vi "temp_Modify Data of First Version.vi"(10 "string":string="V+-V") -> (2 "result string 2":string)   [LabVIEW 2023]
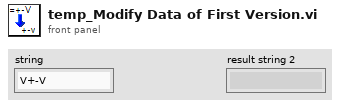
[diagram p1: front panel]
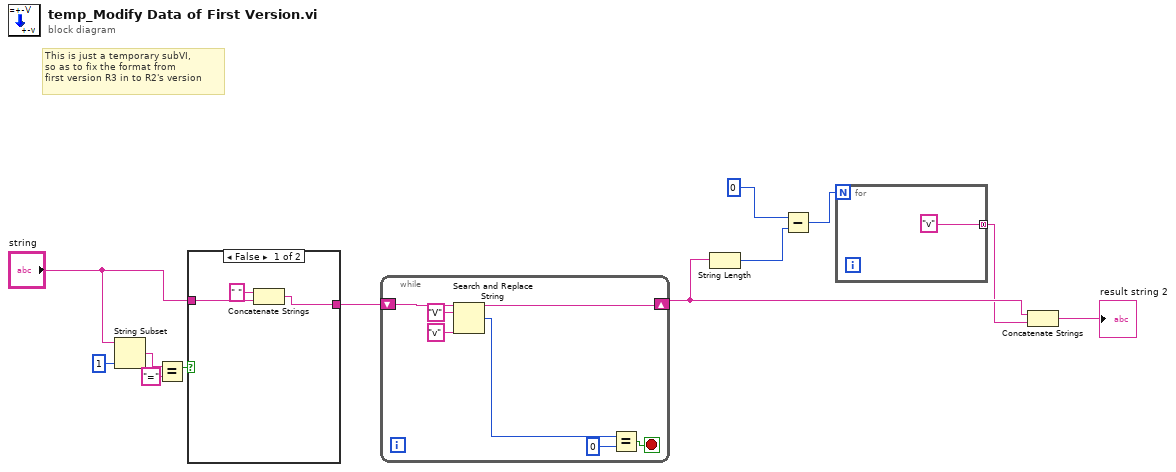
[diagram p0: block diagram]
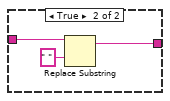
[diagram p2: hidden frame]
diagram:
  # "This is just a temporary subVI,\nso as to fix the format from \nfirst version R3 in to R2's version"
  n1 = String Subset(string="string", length (rest)=1 ("length (rest)")) -> (substring=w9:string)  [unwired: 1 in]
  n2 = Equal?(x=w9, y="=") -> (x = y?=w7:bool)
  n3 = case shown="False" w7 {
    tunnel: [w14 w17] -> w12
    tunnel: "string" -> [w15 w16]
    frame False {
      n4 = Concatenate Strings(" " ("string"), w15) -> (w14:string)
    }
    frame True {
      n5 = Replace Substring(4:" " ("substring (\"\")"), 5:w16) -> (1:w17:string)  [unwired: 2 in, 1 out]
    }
  }
  n6 = while {
    shift-right: [w22] -> w3
    shift-left: w12 -> [w25]
    stop <- w21 stop-if-true
    n7 = Search and Replace String(input string=w25, search string="V", replace string="v" ("replace string (\"\")")) -> (result string=w22:string, number of replacements=w20:i32)  [unwired: 5 in, 2 out]
    n8 = Equal?(x=w20, y=0) -> (x = y?=w21:bool)
  }
  n9 = String Length(string=w3) -> (length=w5:i32)
  n10 = Subtract(x=0, y=w5) -> (x-y=w4:i32)
  n11 = for {
    N: w4 -> [_]
    tunnel: ["v"] -> w2 mode=concatenating
  }
  n12 = Concatenate Strings(w3, w2) -> (→"result string 2":string)
